vi "Write to XML File(string)-mod.vi"(6 "Standalone? (T)":bool=TRUE, 7 "Prompt":string="Select Path to XML File", 8 "error in (no error)":errorcluster, 9 "XML Encoding":string, 10 "XML Input":string, 11 "XML File Path":path) -> (0 "error out":errorcluster, 2 "XML String":string, 3 "XML File Path(duplicate)":path)   [LabVIEW 2020]
doc: "Writes a text string of XML data with accompanying header tags to a text file. Wire data to the <B>XML Input</B> input to determine the polymorphic instance to use or manually select the instance. All XML data must follow the standard LabVIEW XML schema."
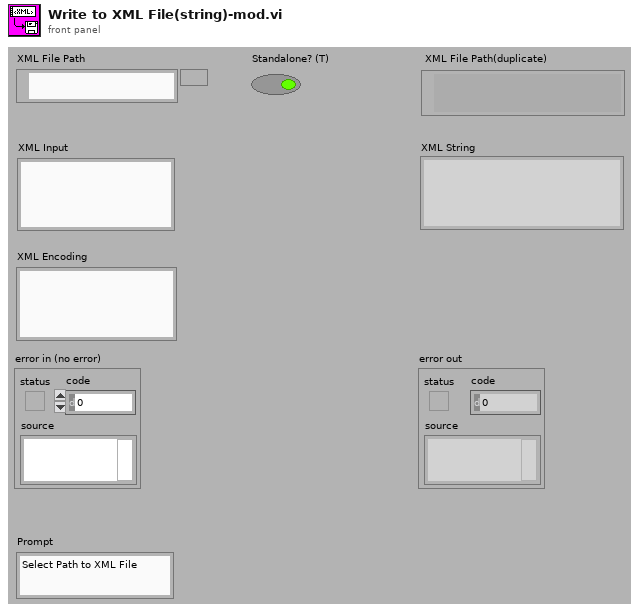
[diagram p1: front panel]
types:
  T1 = enum16{"open", "open or create", "create or replace", "create", "open (read only)"}
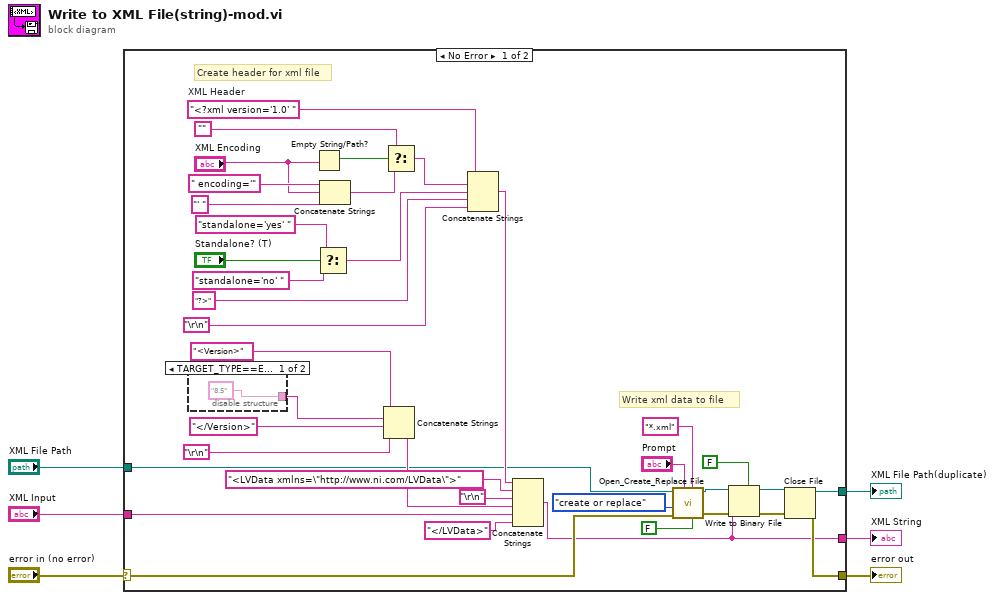
[diagram p0: block diagram]
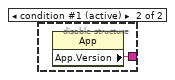
[diagram p2: hidden frame]
diagram:
  n1 = case shown="No Error" "error in (no error)" {
    selector: "error in (no error)" -> [w17 w49]
    tunnel: [w18 w49] -> w5
    tunnel: "XML Input" -> [w29 w48]
    tunnel: [w16 w48] -> w3
    tunnel: [w12 w47] -> w2
    tunnel: "XML File Path" -> [w22 w47]
    frame No Error {
      w44 = "<?xml version='1.0' "  # XML Header
      # "Create header for xml file"
      # "Write xml data to file"
      n2 = disable-structure shown="TARGET_TYPE==Embedded||TARGET_TYPE==PocketPC" {
        disable-tunnel: ["8.5" ("App.Version") w46] -> w27
        frame condition #0 {
        }
        frame condition #1 (active) {
          n3 = property class="App"() -> ("App.Version"=w46:string)  [unwired: 2 in, 2 out]
        }
      }
      n4 = Empty String/Path?(string/path="XML Encoding") -> (empty?=w36:bool)
      n5 = Select(t="standalone='yes' " ("Substring"), s="Standalone? (T)", f="standalone='no' " ("Substring")) -> (s? t:f=w30:string)
      n6 = Concatenate Strings(" encoding='", "XML Encoding", "' " ("Substring")) -> (w35:string)
      n7 = Concatenate Strings("<Version>", w27, "</Version>", "\r\n") -> (w24:string)
      n8 = Select(t="", s=w36, f=w35) -> (s? t:f=w33:string)
      n9 = Concatenate Strings(w44, w33, w30, "?>" ("Substring"), "\r\n") -> (w41:string)
      n10 = Concatenate Strings(w41, "<LVData xmlns=\"http://www.ni.com/LVData\">" ("Substring"), "\r\n", w24, w29, "</LVData>" ("Substring")) -> (w16:string)
      n11 = call <vilib>:"Open_Create_Replace File.vi"("advisory dialog? (display:T)"=FALSE, "pattern"="*.xml", "prompt"="Prompt", "error in (no error)"=w17, "function (open:0)"=T1."create or replace", "file path"=w22) -> ("error out"=w20:errorcluster, "refnum"=w15:refnum<file>)  [unwired: 2 in, 2 out]
      n12 = Write to Binary File(file (use dialog)=w15, data=w16, error in=w20, 5:FALSE ("prepend array or string size? (T)")) -> (refnum out=w13:refnum<file>, error out=w19:errorcluster)  [unwired: 3 out]
      n13 = Close File(refnum=w13, error in=w19) -> (path=w12:path, error out=w18:errorcluster)
    }
    frame Error {
    }
  }
  "error out" <- w5
  "XML String" <- w3
  "XML File Path(duplicate)" <- w2
